vi "Decrement and Saturate to Zero (SubVI).vi"(11 "Data In":u8) -> (3 "Data Out":u8)   [LabVIEW 2015]
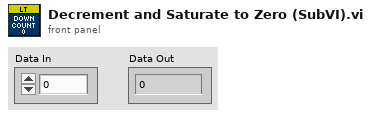
[diagram p1: front panel]
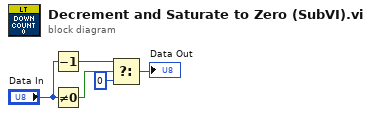
[diagram p0: block diagram]
diagram:
  n1 = Decrement(x="Data In") -> (x-1=w2:u8)
  n2 = Not Equal To 0?(x="Data In") -> (x != 0?=w1:bool)
  n3 = Select(t=w2, s=w1, f=u8 0) -> (s? t:f=→"Data Out":u8)
